vi "FixString.vi"(1 "String":string) -> (0 "Fixed string":string)   [LabVIEW 2014, in "Raspberry Pi Compatible Compiler for LabVIEW.lvlib" / "PythonConfiguration.lvclass"]
uses:
  PythonConfiguration.lvclass
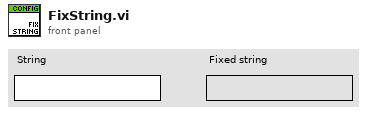
[diagram p1: front panel]
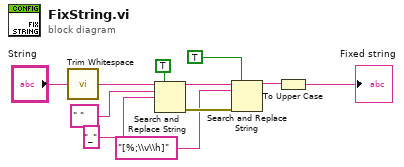
[diagram p0: block diagram]
diagram:
  n1 = call <vilib>:"Trim Whitespace.vi"("string"="String") -> ("trimmed string"=w1:string)  [unwired: 1 in]
  n2 = Search and Replace String(replace all?=TRUE ("replace all? (F)"), input string=w1, search string=" ", replace string="_" ("replace string (\"\")")) -> (result string=w7:string, error out=w6:errorcluster)  [unwired: 4 in, 2 out]
  n3 = Search and Replace String(replace all?=TRUE ("replace all? (F)"), input string=w7, search string="[%;\\v\\h]", error in=w6) -> (result string=w3:string)  [unwired: 4 in, 3 out]
  n4 = To Upper Case(1:w3) -> (0:→"Fixed string":string)
